vi "Read Latest movie role.vi"(8 "error in (no error)":errorcluster, 11 "John Cena in":refnum<class "John Cena.lvclass">) -> (0 "error out":errorcluster, 2 "Latest movie role":string, 3 "John Cena out":refnum<class "John Cena.lvclass">)   [LabVIEW 2019, in "John Cena.lvclass"]
uses:
  John Cena.lvclass
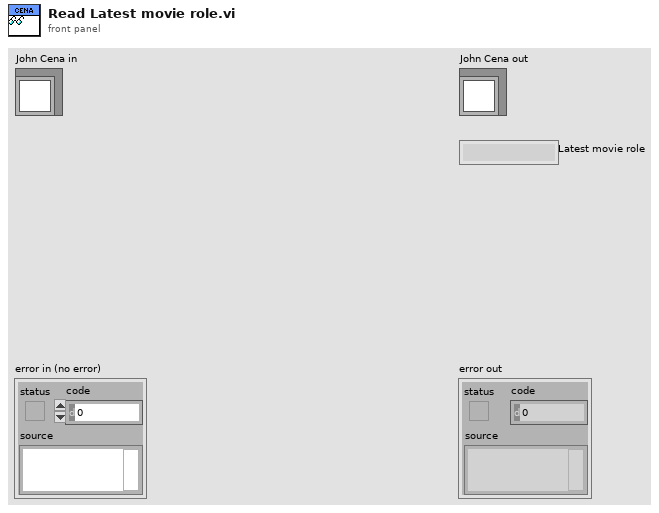
[diagram p1: front panel]
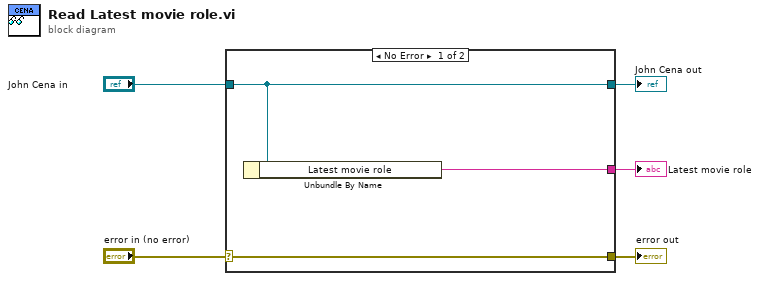
[diagram p0: block diagram]
diagram:
  n1 = case shown="No Error" "error in (no error)" {
    selector: "error in (no error)" -> [w8 w9]
    tunnel: [w8 w9] -> w4
    tunnel: [w7 w10] -> w2
    tunnel: "John Cena in" -> [w7 w10]
    tunnel: [w6 _] -> w1
    frame No Error {
      n2 = Unbundle By Name(w7) -> ("Latest movie role"=w6:string)
    }
    frame Error {
    }
  }
  "error out" <- w4
  "John Cena out" <- w2
  "Latest movie role" <- w1
